vi "diagram2.vi"() -> ()   [LabVIEW 2024]
uses:
  <vilib>/Utility/error.llb/Trim Whitespace One-Sided.vi
  <vilib>/regexp/Match Regular Expression.xnode
  <vilib>/Analysis/NI_AALPro.lvlib
panel:
  out "Array":dbl[](array[numeric])
  out "Densities":dbl[](array[numeric])
  out "Labels":string[](array[string])
  out "Map":map{string, map{string, dbl}}(c390)
  in  "index (row)":i32=2
  out "error":i32
  out "interpolation error":dbl format="%0.2f"
  out "interpolation value":dbl format="%0.2f"
  out "XY Graph":cluster{dbl[], dbl[]}[](graph)
  out "Table Control":string[][](table)
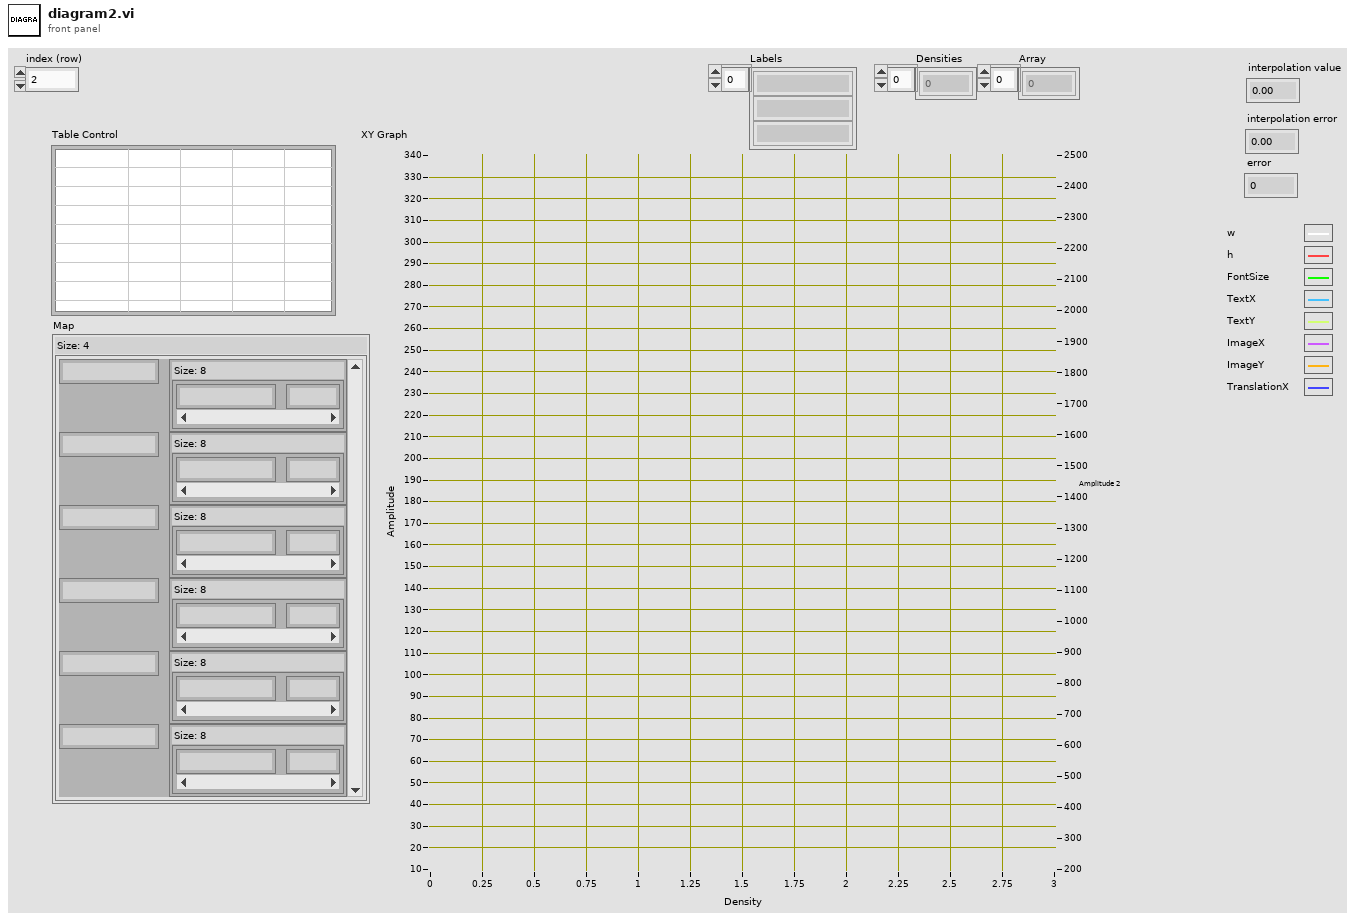
[diagram p1: front panel]
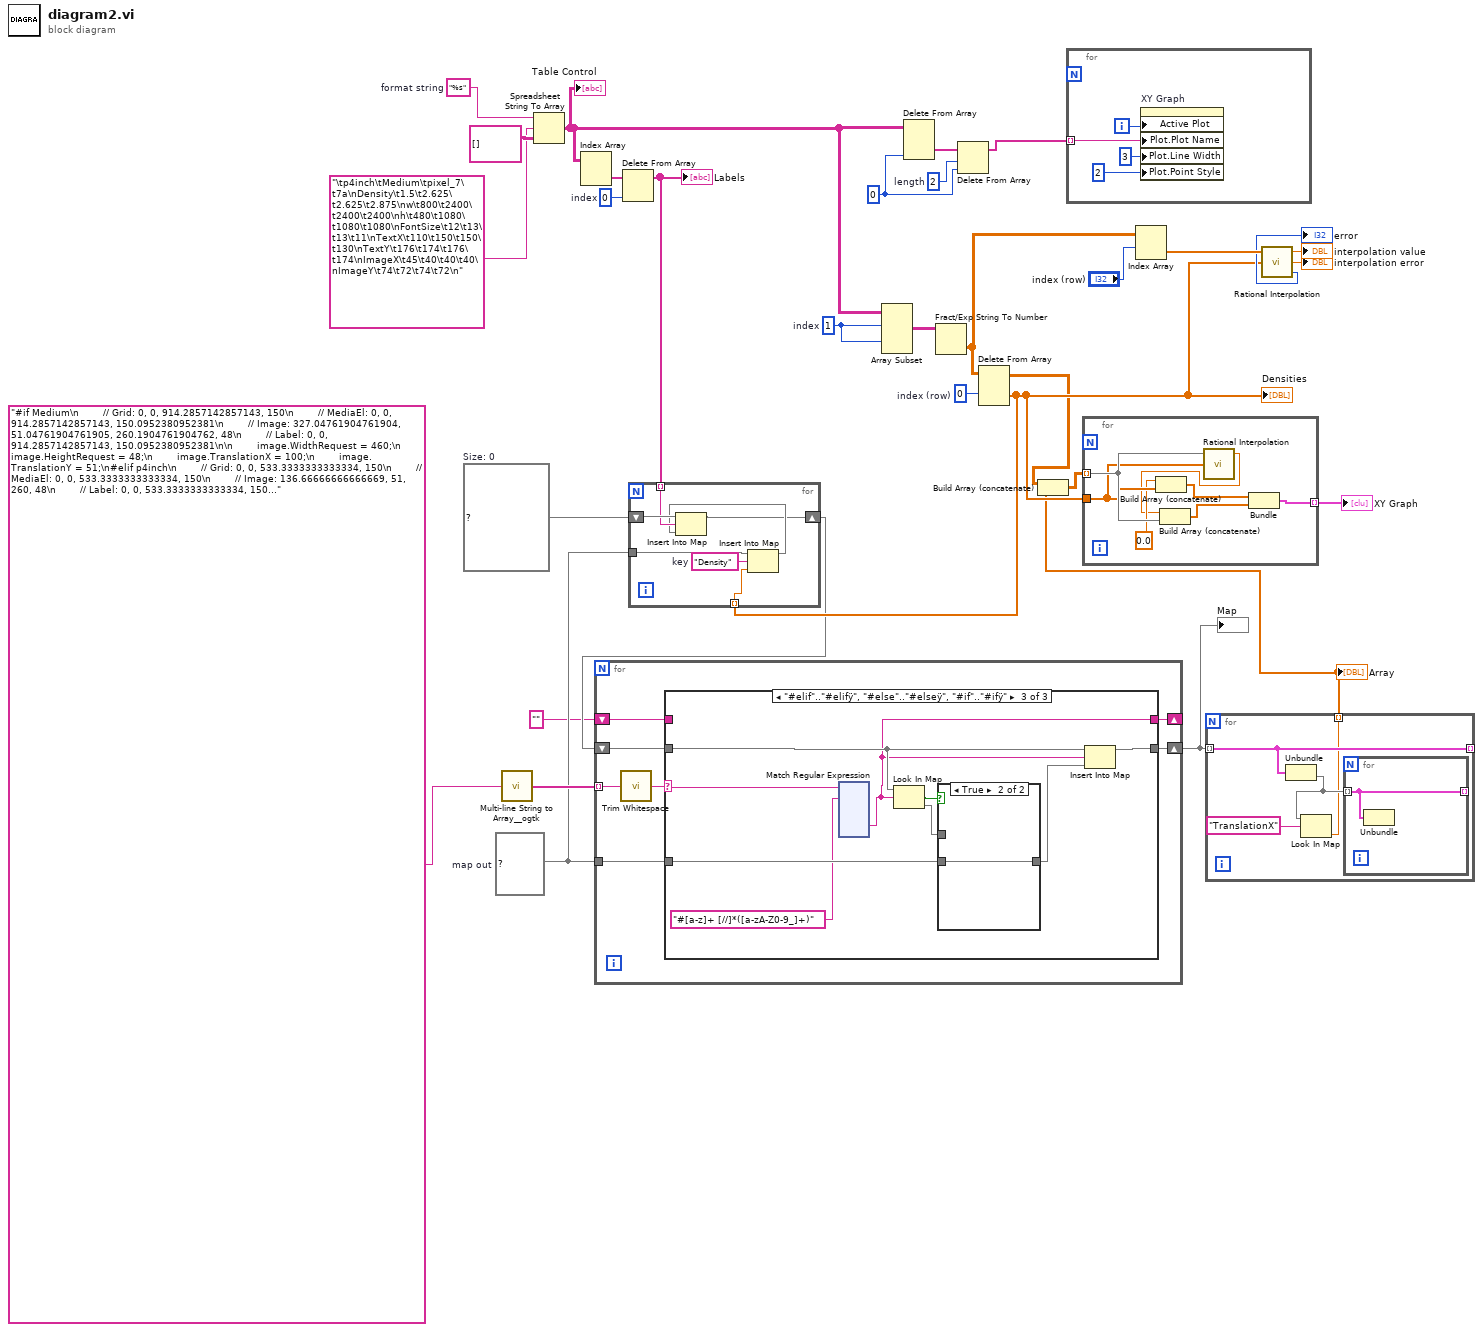
[diagram p0: block diagram]
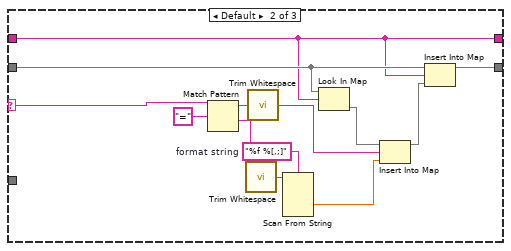
[diagram p3: hidden frame]
diagram:
  w8 = 0  # index
  w17 = "%s"  # format string
  w14 = map{string, map{string, dbl}} {}  # Size: 0
  w11 = map{string, dbl} {}  # map out
  w24 = 2  # length
  w25 = 0
  w30 = 0  # index (row)
  w32 = 1  # index
  n1 = call <userlib>:"Multi-line String to Array__ogtk.vi"("string"="#if Medium\n        // Grid: 0, 0, 914.2857142857143, 150\n        // MediaEl: 0, 0, 914.2857142857143, 150.0952380952381\n        // Image: 327.04761904761904, 51.04761904761905, 260.1904761904762, 48\n        // Label: 0, 0, 914.2857142857143, 150.0952380952381\n\n        image.WidthRequest = 460;\n        image.HeightRequest = 48;\n        image.TranslationX = 100;\n        image.TranslationY = 51;\n#elif p4inch\n        // Grid: 0, 0, 533.3333333333334, 150\n        // MediaEl: 0, 0, 533.3333333333334, 150\n        // Image: 136.66666666666669, 51, 260, 48\n        // Label: 0, 0, 533.3333333333334, 150\n        \n        image.WidthRequest = 260;\n        image.HeightRequest = 48;\n        image.TranslationX = 50;\n        image.TranslationY = 50;\n#elif pixel_7\n        // Grid: 0, 0, 862.4761904761905, 150\n        // MediaEl: 0, 0, 862.4761904761905, 150.0952380952381\n        // Image: 301.1428571428571, 51.04761904761905, 260.1904761904762, 48\n        // Label: 0, 0, 862.4761904761905, 150.0952380952381\n\n        image.WidthRequest = 460;\n        image.HeightRequest = 48;\n        image.TranslationX = 100;\n        image.TranslationY = 50;\n\n#else //7a\n        // Grid:    0, 0, 745.7391304347826, 150\n        // MediaEl: 0, 0, 745.7391304347826, 150.2608695652174\n        // Image:   152.8695652173913, 51.1304347826087, 440, 48\n        // Label:   0, 0, 745.7391304347826, 150.2608695652174\n\n        image.WidthRequest = 440;\n        image.HeightRequest = 48;\n        image.TranslationX = 110;\n        image.TranslationY = 51;\n#endif\n\n#if Medium // 2.625 1080x2400\n            FontSize = 10,\n            TranslationX = 330,\n            TranslationY = 100,\n#elif p4inch //1.5 480x800\n            FontSize = 10, \n            TranslationX = 190,\n            TranslationY = 100,\n#elif pixel_7 // 2.625 1080x2400\n            FontSize = 10,\n            TranslationX = 310,\n            TranslationY = 100,\n#else //7a //2.875 1080x2400\n            FontSize = 10,\n            TranslationX = 280,\n            TranslationY = 100,\n#endif\n") -> ("lines"=w18:string[])
  n2 = Spreadsheet String To Array(format string=w17, spreadsheet string="\tp4inch\tMedium\tpixel_7\t7a\nDensity\t1.5\t2.625\t2.625\t2.875\nw\t800\t2400\t2400\t2400\nh\t480\t1080\t1080\t1080\nFontSize\t12\t13\t13\t11\nTextX\t110\t150\t150\t130\nTextY\t176\t174\t176\t174\nImageX\t45\t40\t40\t40\nImageY\t74\t72\t74\t72\n", array type (2D Dbl)=string[][] []) -> (array=w10:string[][])  [unwired: 1 in]
  "Table Control" <- w10
  n3 = Index Array(array=w10) -> (element=w9:string[])  [unwired: 2 in]
  n4 = Delete From Array(array=w9, index=w8) -> (array with subset deleted=w7:string[])  [unwired: 1 in, 1 out]
  "Labels" <- w7
  n5 = Array Subset(array=w10, index (row)=w32, index (col)=w32) -> (w31:string[][])  [unwired: 2 in]
  n6 = Delete From Array(array=w10, index (col)=w25) -> (deleted portion=w26:string[])  [unwired: 2 in, 1 out]
  n7 = Fract/Exp String To Number(string=w31) -> (number=w29:dbl[][])  [unwired: 3 in, 1 out]
  n8 = Delete From Array(array=w26, length=w24, index=w25) -> (array with subset deleted=w13:string[])  [unwired: 1 out]
  n9 = Delete From Array(array=w29, index (row)=w30) -> (deleted portion=w12:dbl[], array with subset deleted=w3:dbl[][])  [unwired: 2 in]
  "Densities" <- w12
  n10 = for {
    tunnel: w7 -> [w38] mode=indexing
    tunnel: w12 -> [w37] mode=indexing
    tunnel: w11 -> [w35]
    shift-right: [w33] -> w6
    shift-left: w14 -> [w39]
    w36 = "Density"  # key
    n11 = Insert Into Map(map in=w35, key=w36, value=w37) -> (map out=w34:map{string, dbl})  [unwired: 2 out]
    n12 = Insert Into Map(map in=w39, key=w38, value=w34) -> (map out=w33:map{string, map{string, dbl}})  [unwired: 2 out]
  }
  n13 = for {
    tunnel: w18 -> [w46] mode=indexing
    shift-right: [w44] -> w4
    shift-left: w6 -> [w45]
    tunnel: w11 -> [w43]
    shift-right: [w42] -> _
    shift-left: "" ("submatch 1") -> [w41]
    n14 = call <vilib>:"Trim Whitespace.vi"("string"=w46) -> ("trimmed string"=w40:string)  [unwired: 1 in]
    n15 = case shown="\"#elif\"..\"#elifÿ\", \"#else\"..\"#elseÿ\", \"#if\"..\"#ifÿ\"" w40 {
      selector: w40 -> [_ w51 w64]
      tunnel: w45 -> [w48 w56 w66]
      tunnel: [w48 w55 w70] -> w44
      tunnel: w43 -> [_ _ w67]
      tunnel: [w47 w53 w62] -> w42
      tunnel: w41 -> [w47 w53 _]
      frame "", "#endif", "//".."//ÿ" {
      }
      frame Default {
        w60 = "%f %[,;]"  # format string
        n16 = Match Pattern(string=w51, regular expression="=" ("search string/char (-)")) -> (before substring=w50:string, after substring=w49:string)  [unwired: 1 in, 2 out]
        n17 = call <vilib>:"Trim Whitespace.vi"("string"=w49) -> ("trimmed string"=w61:string)  [unwired: 1 in]
        n18 = call <vilib>:"Trim Whitespace.vi"("string"=w50) -> ("trimmed string"=w59:string)  [unwired: 1 in]
        n19 = Scan From String(format string=w60, input string=w61) -> (output 1=w58:dbl)  [unwired: 5 in, 3 out]
        n20 = Look In Map(map=w56, key=w53) -> (value=w57:map{string, dbl})  [unwired: 1 in, 1 out]
        n21 = Insert Into Map(map in=w57, key=w59, value=w58) -> (map out=w54:map{string, dbl})  [unwired: 2 out]
        n22 = Insert Into Map(map in=w56, key=w53, value=w54) -> (map out=w55:map{string, map{string, dbl}})  [unwired: 2 out]
      }
      frame "#elif".."#elifÿ", "#else".."#elseÿ", "#if".."#ifÿ" {
        n23 = xnode "Match Regular Expression"("input string"=w64, "regular expression"="#[a-z]+ [//]*([a-zA-Z0-9_]+)" ("search string/char (-)")) -> ("submatch 1"=w62:string)  [unwired: 4 in, 6 out]
        n24 = Look In Map(map=w66, key=w62) -> (key not found?=w69:bool, value=w65:map{string, dbl})  [unwired: 1 in]
        n25 = case shown="True" w69 {
          tunnel: [w191 w192] -> w68
          tunnel: w67 -> [_ w192]
          tunnel: w65 -> [w191 _]
          frame False {
          }
          frame True {
          }
        }
        n26 = Insert Into Map(map in=w66, key=w62, value=w68) -> (map out=w70:map{string, map{string, dbl}})  [unwired: 2 out]
      }
    }
  }
  "Map" <- w4
  n27 = for {
    tunnel: w13 -> [w195] mode=indexing
    i -> [w196]
    n28 = property on="XY Graph" class="XYGraph (strict)"("Active Plot"=w196, "Plot.Plot Name"=w195, "Plot.Line Width"=u8 3, "Plot.Point Style"=u8 2) -> ()  [unwired: 2 in, 2 out]
  }
  n29 = Index Array(array=w29, index (row)="index (row)") -> (element=w23:dbl[])  [unwired: 1 in]
  n30 = for {
    tunnel: [w200] -> _ mode=indexing
    tunnel: w4 -> [w200] mode=indexing
    tunnel: [w197] -> w2 mode=indexing
    n31 = Unbundle(w200) -> ("map out"=w199:map{string, dbl})  [unwired: 1 out]
    n32 = Look In Map(map=w199, key="TranslationX" ("trimmed string")) -> (value=w197:dbl)  [unwired: 1 in, 1 out]
    n33 = for {
      tunnel: [w201] -> _ mode=indexing
      tunnel: w199 -> [w201] mode=indexing
      n34 = Unbundle(w201) -> ()  [unwired: 2 out]
    }
  }
  "Array" <- w2
  n35 = Build Array (concatenate)(w3, w2) -> (w1:dbl[][])
  n36 = for {
    tunnel: w1 -> [w207] mode=indexing
    tunnel: w12 -> [w204]
    tunnel: [w208] -> w27 mode=indexing
    n37 = Build Array (concatenate)(0.0, w204) -> (w205:dbl[])
    n38 = call <vilib>:"Rational Interpolation.vi"("X"=w204, "Y"=w207) -> ("interpolation value"=w202:dbl)  [unwired: 1 in, 2 out]
    n39 = Build Array (concatenate)(w202, w207) -> (w206:dbl[])
    n40 = Bundle(w205, w206) -> (w208:cluster{dbl[], dbl[]})  [unwired: 1 in]
  }
  "XY Graph" <- w27
  n41 = call <vilib>:"Rational Interpolation.vi"("X"=w12, "Y"=w23) -> ("error"=→"error":i32, "interpolation error"=→"interpolation error":dbl, "interpolation value"=→"interpolation value":dbl)  [unwired: 1 in]
